vi "HGET.vi"(8 "error in (no error)":errorcluster, 9 "field":string, 10 "key":string, 11 "Redis Client in":refnum<class "Redis Client.lvclass">) -> (0 "error out":errorcluster, 1 "found?":bool, 2 "RESP3 Value":variant, 3 "Redis Client out":refnum<class "Redis Client.lvclass">)   [LabVIEW 2019, in "Redis Client for LabVIEW.lvlib" / "Redis Client.lvclass"]
uses:
  Redis Client.lvclass
  lib/RESP3-for-LabVIEW/RESP3/subVIs/RESP3 Make String Base.vi
  lib/RESP3-for-LabVIEW/RESP3/types/RESP3 data type attribute.vi
  lib/RESP3-for-LabVIEW/RESP3/RESP3.lvlib
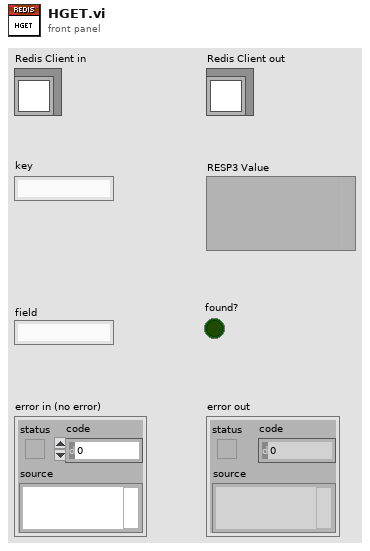
[diagram p1: front panel]
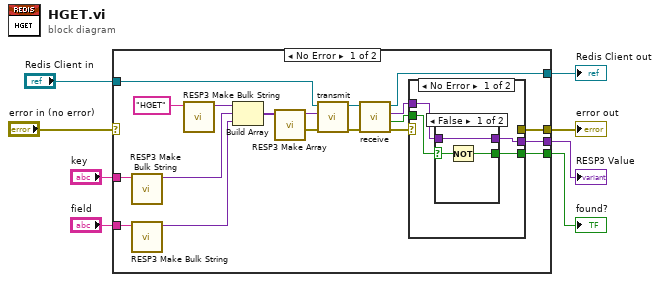
[diagram p0: block diagram]
diagram:
  n1 = case shown="No Error" "error in (no error)" {
    selector: "error in (no error)" -> [_ w37]
    tunnel: [w13 w37] -> w7
    tunnel: "Redis Client in" -> [w27 w36]
    tunnel: [w24 w36] -> w5
    tunnel: "key" -> [w21 _]
    tunnel: "field" -> [w20 _]
    tunnel: [w12 _] -> w2
    tunnel: [w9 _] -> w1
    frame No Error {
      n2 = call "RESP3 Make Bulk String.vi"("String"=w21) -> ("RESP3 Value out"=w18:variant)  [unwired: 9 in, 1 out]
      n3 = call "RESP3 Make Bulk String.vi"("String"=w20) -> ("RESP3 Value out"=w17:variant)  [unwired: 9 in, 1 out]
      n4 = call "RESP3 Make Bulk String.vi"("String"="HGET" ("string in")) -> ("RESP3 Value out"=w19:variant)  [unwired: 9 in, 1 out]
      n5 = Build Array(w19, w18, w17) -> (w26:variant[])
      n6 = call "RESP3 Make Array.vi"("RESP3 Values in"=w26) -> ("error out"=w15:errorcluster, "RESP3 Value out"=w16:variant)  [unwired: 9 in]
      n7 = call-dynamic "transmit.vi"("error in (no error)"=w15, "RESP3 Value"=w16, "Redis Client in"=w27) -> ("error out"=w23:errorcluster, "Redis Client out"=w25:refnum<class "Redis Client.lvclass">)  [unwired: 7 in]
      n8 = call-dynamic "receive.vi"("error in (no error)"=w23, "Redis Client in"=w25) -> ("error out"=w11:errorcluster, "timed out?"=w10:bool, "RESP3 Value"=w14:variant, "Redis Client out"=w24:refnum<class "Redis Client.lvclass">)  [unwired: 6 in]
      n9 = case shown="No Error" w11 {
        selector: w11 -> [_ w35]
        tunnel: w14 -> [w31 _]
        tunnel: [_ w35] -> w13
        tunnel: [w30 _] -> w12
        tunnel: w10 -> [w29 _]
        tunnel: [w28 _] -> w9
        frame No Error {
          n10 = case shown="False" w29 {
            selector: w29 -> [w32 _]
            tunnel: w31 -> [w33 _]
            tunnel: [w34 _] -> w30
            tunnel: [w33 _] -> w28
            frame False {
              n11 = Not(x=w32) -> (.not. x?=w34:bool)
            }
            frame True {
            }
          }
        }
        frame Error {
        }
      }
    }
    frame Error {
    }
  }
  "error out" <- w7
  "Redis Client out" <- w5
  "RESP3 Value" <- w1
  "found?" <- w2
